vi "NextMove.vi"(8 "error in (no error)":errorcluster, 10 "Point":cluster{"X":dbl, "Y":dbl}, 11 "OccupancyMap in":refnum<class "OccupancyMap.lvclass">) -> (0 "error out":errorcluster, 2 "NextMove":cluster{"X":dbl, "Y":dbl}[](array[cluster]), 3 "OccupancyMap out":refnum<class "OccupancyMap.lvclass">)   [LabVIEW 2010, in "OccupancyMap.lvclass"]
uses:
  OccupancyMap.lvclass
  OccupancyMap.lvclass/OccupancyMap.ctl
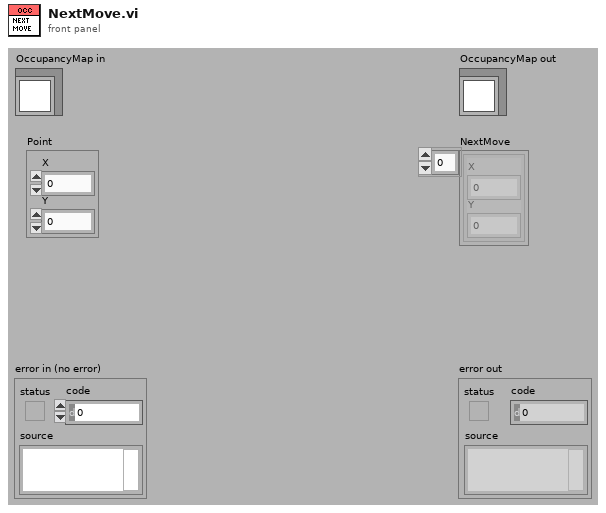
[diagram p1: front panel]
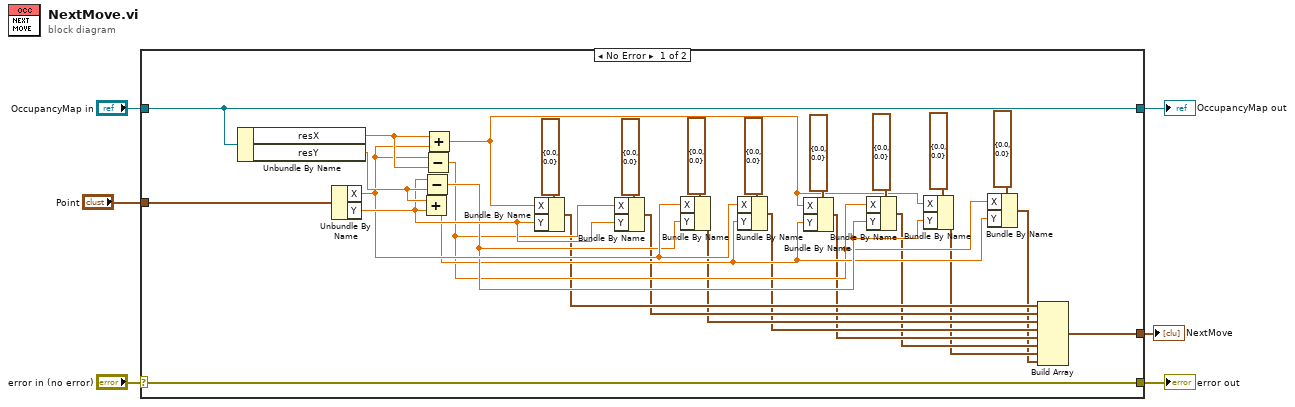
[diagram p0: block diagram]
diagram:
  n1 = case shown="No Error" "error in (no error)" {
    selector: "error in (no error)" -> [w34 w36]
    tunnel: [w34 w36] -> w5
    tunnel: [w25 w35] -> w3
    tunnel: "OccupancyMap in" -> [w25 w35]
    tunnel: "Point" -> [w24 _]
    tunnel: [w7 _] -> w1
    frame No Error {
      n2 = Unbundle By Name(w25) -> ("resX"=w32:dbl, "resY"=w33:dbl)
      n3 = Unbundle By Name(w24) -> ("X"=w26:dbl, "Y"=w29:dbl)
      n4 = Add(x=w33, y=w29) -> (x+y=w17:dbl)
      n5 = Subtract(x=w29, y=w33) -> (x-y=w19:dbl)
      n6 = Subtract(x=w26, y=w32) -> (x-y=w16:dbl)
      n7 = Add(x=w32, y=w26) -> (x+y=w20:dbl)
      n8 = Bundle By Name(cluster=cluster{"X":dbl, "Y":dbl} {"X"=0.0, "Y"=0.0}, "X"=w20, "Y"=w29) -> (w15:cluster{"X":dbl, "Y":dbl})
      n9 = Bundle By Name(cluster=cluster{"X":dbl, "Y":dbl} {"X"=0.0, "Y"=0.0}, "X"=w16, "Y"=w29) -> (w14:cluster{"X":dbl, "Y":dbl})
      n10 = Bundle By Name(cluster=cluster{"X":dbl, "Y":dbl} {"X"=0.0, "Y"=0.0}, "X"=w26, "Y"=w19) -> (w13:cluster{"X":dbl, "Y":dbl})
      n11 = Bundle By Name(cluster=cluster{"X":dbl, "Y":dbl} {"X"=0.0, "Y"=0.0}, "X"=w26, "Y"=w17) -> (w12:cluster{"X":dbl, "Y":dbl})
      n12 = Bundle By Name(cluster=cluster{"X":dbl, "Y":dbl} {"X"=0.0, "Y"=0.0}, "X"=w20, "Y"=w17) -> (w11:cluster{"X":dbl, "Y":dbl})
      n13 = Bundle By Name(cluster=cluster{"X":dbl, "Y":dbl} {"X"=0.0, "Y"=0.0}, "X"=w16, "Y"=w19) -> (w10:cluster{"X":dbl, "Y":dbl})
      n14 = Bundle By Name(cluster=cluster{"X":dbl, "Y":dbl} {"X"=0.0, "Y"=0.0}, "X"=w20, "Y"=w19) -> (w9:cluster{"X":dbl, "Y":dbl})
      n15 = Bundle By Name(cluster=cluster{"X":dbl, "Y":dbl} {"X"=0.0, "Y"=0.0}, "X"=w16, "Y"=w17) -> (w8:cluster{"X":dbl, "Y":dbl})
      n16 = Build Array(w15, w14, w13, w12, w11, w10, w9, w8) -> (w7:cluster{"X":dbl, "Y":dbl}[])
    }
    frame Error {
    }
  }
  "error out" <- w5
  "OccupancyMap out" <- w3
  "NextMove" <- w1
